vi "Create Core.vi"(8 "error in (no error)":errorcluster, 11 "Core Component in":refnum<class "Core Component.lvclass">) -> (0 "error out":errorcluster, 3 "Core Component out":refnum<class "Core Component.lvclass">)   [LabVIEW 2017, in "DSF Core.lvlib" / "Core Component.lvclass"]
uses:
  Core Component.lvclass
  C:/Git/DSF/Core/Classes/Component/Component.lvclass
  User Interface/Core/Core User Interfaces.lvclass
  C:/Git/DSF/Core/Classes/Component User Interface/Component User Interfaces.lvclass
  Configuration/Core/Core Configurations.lvclass
  C:/Git/DSF/Core/Classes/Component Configuration/Component Configurations.lvclass
  Component.lvclass
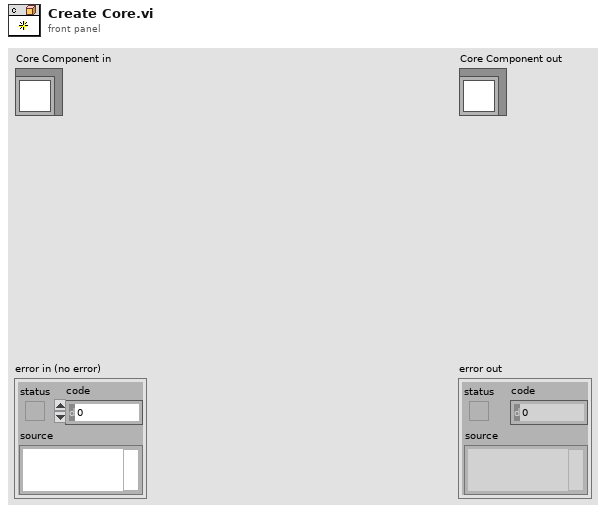
[diagram p1: front panel]
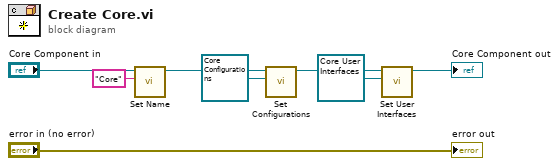
[diagram p0: block diagram]
diagram:
  n1 = call "Set Name.vi"("name"="Core", "Component in"="Core Component in") -> ("Component out"=w6:refnum<class "Core Component.lvclass">)  [unwired: 9 in]
  n2 = call "Set Configurations.vi"("Configurations"=refnum<class "Core Configurations.lvclass"> refnum ("DSF Core.lvlib:Core Configurations.lvclass"), "Component in"=w6) -> ("Component out"=w5:refnum<class "Core Component.lvclass">)  [unwired: 9 in]
  n3 = call "Set User Interfaces.vi"("User Interfaces"=refnum<class "Core User Interfaces.lvclass"> refnum ("DSF Core.lvlib:Core User Interfaces.lvclass"), "Component in"=w5) -> ("Component out"=→"Core Component out":refnum<class "Core Component.lvclass">)  [unwired: 9 in]
  "error out" <- "error in (no error)"
